vi "Get User Access Level.vi"(8 "error in (no error)":errorcluster, 10 "Username":string, 11 "UserPwd DB in":refnum<class "UserPwd DB.lvclass">) -> (0 "error out":errorcluster, 1 "Access":T1, 2 "found":bool, 3 "UserPwd DB out":refnum<class "UserPwd DB.lvclass">, 4 "Array of Permissions":bool[](array[boolean]))   [LabVIEW 2016, in "UserPwd DB.lvlib" / "UserPwd DB.lvclass"]
uses:
  <userlib>/Common Components/UserPwd DB/UserPwd DB/UserPwd DB.lvclass
  <userlib>/Common Components/UserPwd DB/UserPwd DB/Access Level.ctl
  <userlib>/Common Components/UserPwd DB/UserPwd DB/UserPwd DB.lvclass/UserPwd DB.ctl
  <userlib>/Common Components/UserPwd DB/UserPwd DB/Data saved.ctl
  <vilib>/addons/_JKI.lib/Serialization/JSON/JKI JSON Serialization.lvlib
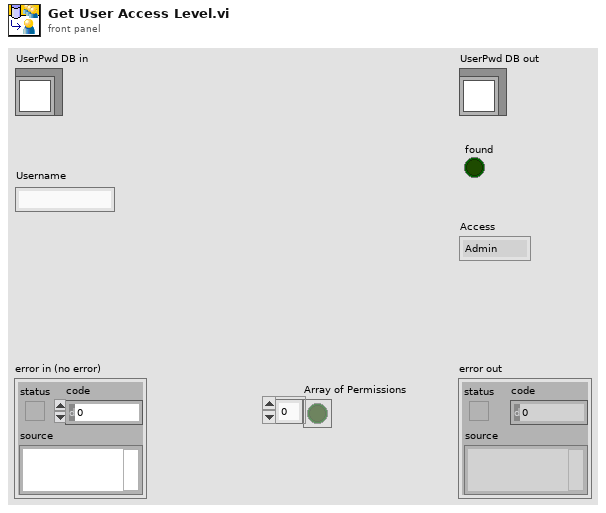
[diagram p1: front panel]
types:
  T1 = typedef "UserPwd DB.lvlib/UserPwd DB.lvclass/Access Level.ctl" = enum16{"Admin", "User lv1", "User lv2", "User lv3", "User lv4", "User lv5", "User lv6", "User lv7", "User lv8", "User lv9", "Guest"}
  T2 = typedef "UserPwd DB.lvlib/UserPwd DB.lvclass/Data saved.ctl" = cluster{"Encrypted Password":string, "Access":T1, "Permission":u32}
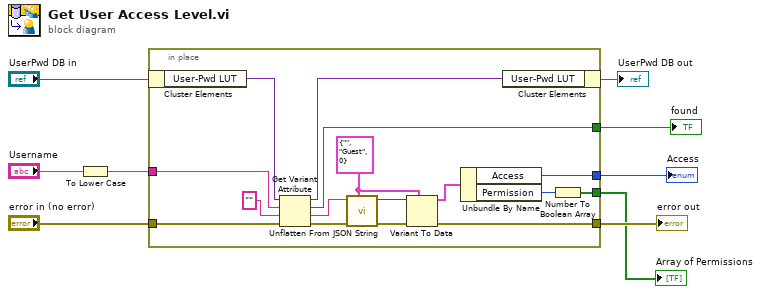
[diagram p0: block diagram]
diagram:
  n1 = To Lower Case(string="Username") -> (all lower case string=w2:string)
  n2 = in-place {
    in-place-border: w2 -> [w23]
    in-place-border: "error in (no error)" -> [w22]
    in-place-border: [w15] -> w5
    in-place-border: [w20] -> w4
    in-place-border: [w19] -> w3
    in-place-border: [w10] -> w1
    w13 = T2 {"Encrypted Password"="", "Access"=enum."Guest", "Permission"=0} ("Data")
    n3 = in-place-cluster #1("UserPwd DB in") -> ("User-Pwd LUT"=w25:variant)
    n4 = Get Variant Attribute(Variant=w25, name=w23, default value (empty Variant)="" ("Password"), error in=w22) -> (duplicate Variant=w24:variant, found=w19:bool, value=w16:string, error out=w21:errorcluster)
    n5 = call <vilib>:"Unflatten From JSON String.vi"("Type and Defaults"=w13, "error in (no error)"=w21, "JSON String"=w16) -> ("error out"=w17:errorcluster, "Variant"=w14:variant)  [unwired: 7 in]
    n6 = Variant To Data(error in=w17, type=w13, Variant=w14) -> (data=w12:T2, error out=w15:errorcluster)
    n7 = Unbundle By Name(w12) -> ("Access"=w20:T1, "Permission"=w11:u32)
    n8 = in-place-cluster #1("User-Pwd LUT"=w24) -> (→"UserPwd DB out":refnum<class "UserPwd DB.lvclass">)
    n9 = Number To Boolean Array(number=w11) -> (Boolean array=w10:bool[])
  }
  "error out" <- w5
  "Access" <- w4
  "found" <- w3
  "Array of Permissions" <- w1
